vi "INR.vi"(1 "Port":refnum<visa-resource-name>="COM4" caption="VISA 리소스 이름", 2 "baud rate (9600)":u32=115200 caption="보 전송속도(9600)") -> (0 "InPOS (X)":bool, 3 "VISA out":refnum<visa-resource-name>, 4 "InPOS (Y)":bool, 5 "Limit+  (X)":bool, 6 "Limit+ (Y)":bool, 7 "Limit-  (X)":bool, 8 "Limit- (Y)":bool, 9 "HOMing  (X)":bool, 10 "HOMing(Y)":bool, 11 "RUN  (X)":bool, 12 "INR Information(X)":string, 13 "INR Information(Y)":string, 14 "Error Out":errorcluster caption="에러 출력", 15 "RUN (Y)":bool)   [LabVIEW 2010]
uses:
  <vilib>/Instr/_visa.llb/VISA Flush IO Buffer Mask.ctl
  <vilib>/Instr/_visa.llb/VISA Configure Serial Port (Instr).vi
panel:
  out "Status Y":bool[](array[boolean])
  out "Status X":bool[](array[boolean])
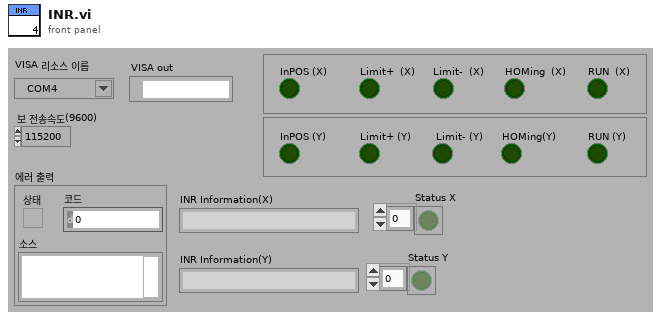
[diagram p1: front panel]
types:
  T1 = typedef "VISA Flush IO Buffer Mask.ctl" = u16
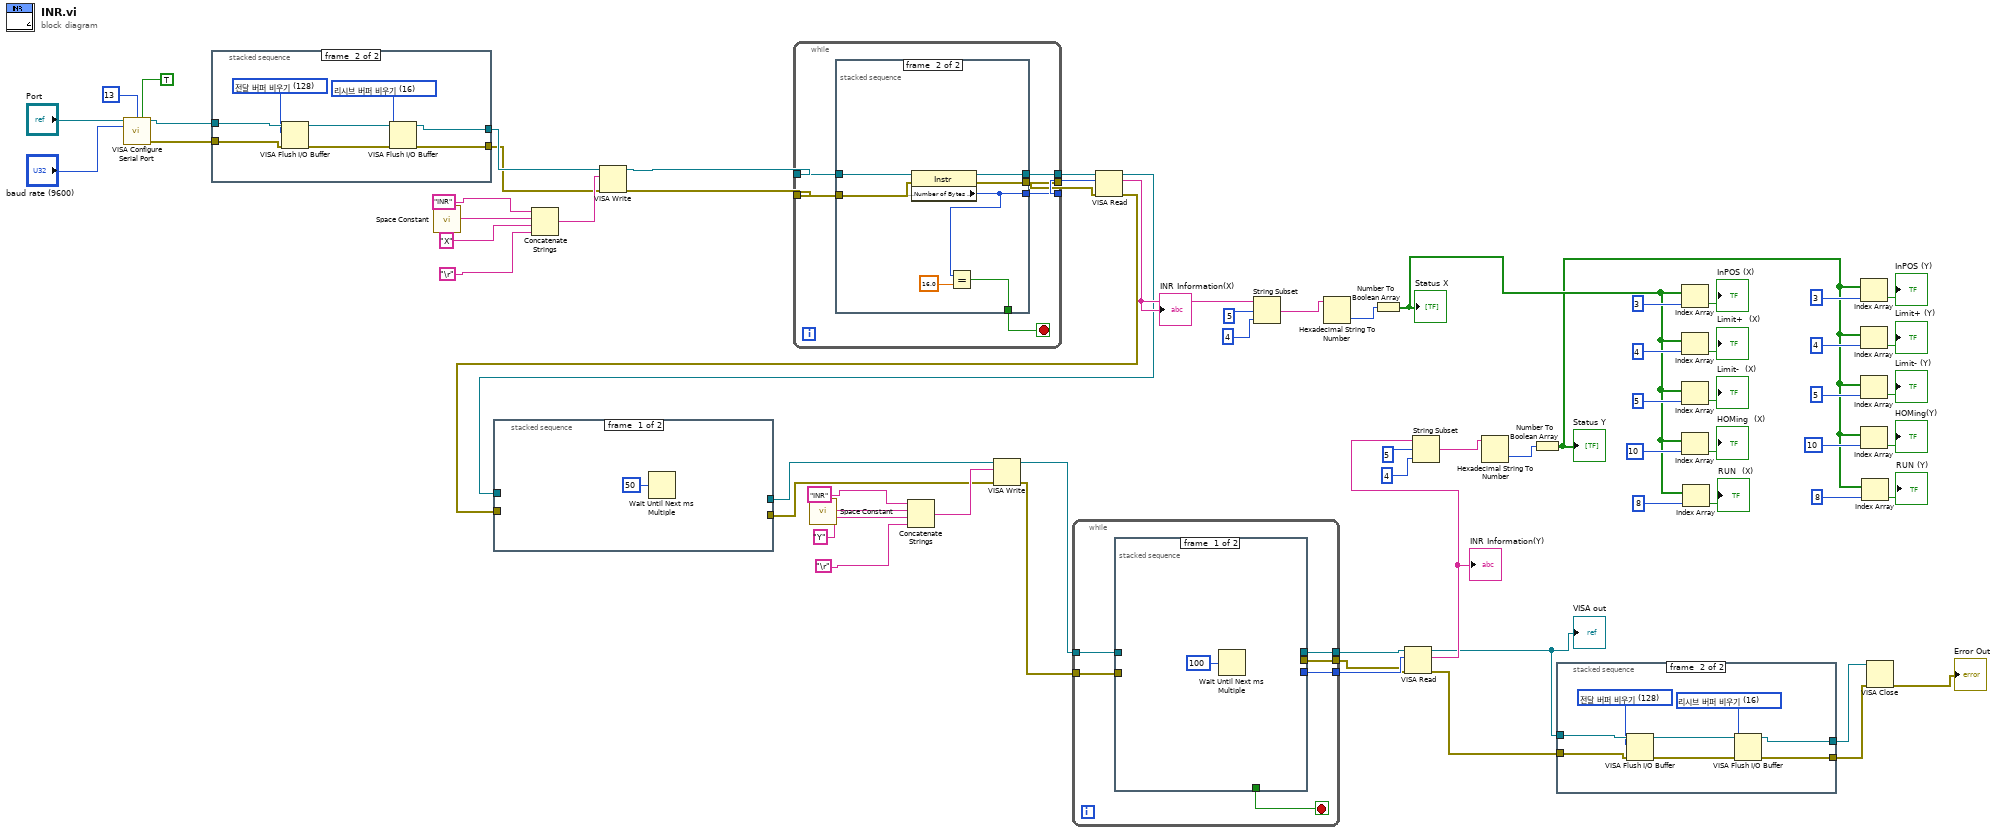
[diagram p0: block diagram]
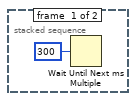
[diagram p2: hidden frame]
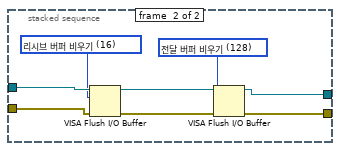
[diagram p3: hidden frame]
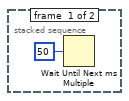
[diagram p4: hidden frame]
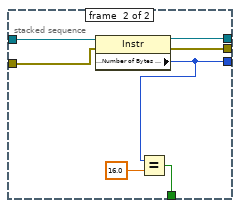
[diagram p5: hidden frame]
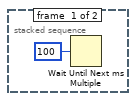
[diagram p6: hidden frame]
diagram:
  n1 = call-poly "VISA Configure Serial Port"("VISA resource name"="Port", "termination char\n(0xA = '\\n' = LF)"=i16 13 ("termination char\n(0xA = '\\n' = LF)"), "Enable Termination\nChar (T)"=TRUE ("Enable Termination\nChar (T)"), "baud rate (9600)"="baud rate (9600)") -> ("VISA resource name out"=w34:refnum<visa-resource-name>, "error out"=w33:errorcluster)  [unwired: 10 in]
  n2 = stacked-sequence {
    tunnel: w34 -> [_ w78]
    tunnel: w33 -> [_ w77]
    tunnel: [_ w73] -> w32
    tunnel: [_ w72] -> w31
    frame #0 {
      n3 = Wait Until Next ms Multiple(millisecond multiple=u32 50 ("ms 배수")) -> ()  [unwired: 1 out]
    }
    frame #1 {
      w71 = T1 16 items=["리시브 버퍼 비우기"=16, "전달 버퍼 디바이스에 쓰기"=32, "리시브 버퍼 비우기(I/O 없음)"=64, "전달 버퍼 비우기"=128] ("Mask")
      w76 = T1 128 items=["리시브 버퍼 비우기"=16, "전달 버퍼 디바이스에 쓰기"=32, "리시브 버퍼 비우기(I/O 없음)"=64, "전달 버퍼 비우기"=128] ("Mask")
      n4 = VISA Flush I/O Buffer(VISA resource name=w78, mask (16)=w76, error in (no error)=w77) -> (VISA resource name out=w75:refnum<visa-resource-name>, error out=w74:errorcluster)
      n5 = VISA Flush I/O Buffer(VISA resource name=w75, mask (16)=w71, error in (no error)=w74) -> (VISA resource name out=w73:refnum<visa-resource-name>, error out=w72:errorcluster)
    }
  }
  n6 = call <vilib>:"Space Constant.vi"() -> ("String"=w67:string)
  n7 = Concatenate Strings("INR", w67, "X", "\r") -> (w68:string)
  n8 = VISA Write(VISA resource name=w32, write buffer=w68, error in (no error)=w31) -> (VISA resource name out=w62:refnum<visa-resource-name>, error out=w61:errorcluster)  [unwired: 1 out]
  n9 = while {
    tunnel: w62 -> [w84]
    tunnel: w61 -> [w83]
    tunnel: [w82] -> w66
    tunnel: [w80] -> w65
    tunnel: [w81] -> w64
    stop <- w79 stop-if-true
    n10 = stacked-sequence {
      tunnel: w84 -> [_ w92]
      tunnel: w83 -> [_ w91]
      tunnel: [_ w90] -> w82
      tunnel: [_ w89] -> w81
      tunnel: [_ w87] -> w80
      tunnel: [_ w86] -> w79
      frame #0 {
        n11 = Wait Until Next ms Multiple(millisecond multiple=u32 100 ("대기 시간(ms)")) -> ()  [unwired: 1 out]
      }
      frame #1 {
        n12 = property class="Instr"(reference=w92, error in=w91) -> (reference out=w90:refnum<visa-resource-name>, error out=w89:errorcluster, "Serial Settings:Number of Bytes at Serial Port"=w87:u32)
        n13 = Equal?(x=w87, y=16.0) -> (x = y?=w86:bool)
      }
    }
  }
  n14 = call <vilib>:"Space Constant.vi"() -> ("String"=w59:string)
  n15 = Concatenate Strings("INR", w59, "Y", "\r") -> (w57:string)
  n16 = VISA Read(VISA resource name=w66, byte count=w65, error in (no error)=w64) -> (VISA resource name out=w28:refnum<visa-resource-name>, read buffer=w51:string, error out=w27:errorcluster)  [unwired: 1 out]
  "INR Information(X)" <- w51
  n17 = stacked-sequence {
    tunnel: w28 -> [_ w101]
    tunnel: w27 -> [_ w100]
    tunnel: [_ w96] -> w30
    tunnel: [_ w95] -> w29
    frame #0 {
      n18 = Wait Until Next ms Multiple(millisecond multiple=u32 50 ("ms 배수")) -> ()  [unwired: 1 out]
    }
    frame #1 {
      w94 = T1 128 items=["리시브 버퍼 비우기"=16, "전달 버퍼 디바이스에 쓰기"=32, "리시브 버퍼 비우기(I/O 없음)"=64, "전달 버퍼 비우기"=128] ("Mask")
      w99 = T1 16 items=["리시브 버퍼 비우기"=16, "전달 버퍼 디바이스에 쓰기"=32, "리시브 버퍼 비우기(I/O 없음)"=64, "전달 버퍼 비우기"=128] ("Mask")
      n19 = VISA Flush I/O Buffer(VISA resource name=w101, mask (16)=w99, error in (no error)=w100) -> (VISA resource name out=w98:refnum<visa-resource-name>, error out=w97:errorcluster)
      n20 = VISA Flush I/O Buffer(VISA resource name=w98, mask (16)=w94, error in (no error)=w97) -> (VISA resource name out=w96:refnum<visa-resource-name>, error out=w95:errorcluster)
    }
  }
  n21 = VISA Write(VISA resource name=w30, write buffer=w57, error in (no error)=w29) -> (VISA resource name out=w56:refnum<visa-resource-name>, error out=w55:errorcluster)  [unwired: 1 out]
  n22 = while {
    tunnel: w56 -> [w107]
    tunnel: w55 -> [w106]
    tunnel: [w105] -> w54
    tunnel: [w103] -> w53
    tunnel: [w104] -> w52
    stop <- w102 stop-if-true
    n23 = stacked-sequence {
      tunnel: w107 -> [_ w115]
      tunnel: w106 -> [_ w114]
      tunnel: [_ w113] -> w105
      tunnel: [_ w112] -> w104
      tunnel: [_ w110] -> w103
      tunnel: [_ w109] -> w102
      frame #0 {
        n24 = Wait Until Next ms Multiple(millisecond multiple=u32 100 ("대기 시간(ms)")) -> ()  [unwired: 1 out]
      }
      frame #1 {
        n25 = property class="Instr"(reference=w115, error in=w114) -> (reference out=w113:refnum<visa-resource-name>, error out=w112:errorcluster, "Serial Settings:Number of Bytes at Serial Port"=w110:u32)
        n26 = Equal?(x=w110, y=16.0) -> (x = y?=w109:bool)
      }
    }
  }
  n27 = String Subset(string=w51, offset (0)=5 ("오프셋(0)"), length (rest)=4 ("길이(나머지)")) -> (substring=w46:string)
  n28 = Hexadecimal String To Number(string=w46) -> (number=w45:u32)  [unwired: 2 in, 1 out]
  n29 = Number To Boolean Array(number=w45) -> (Boolean array=w12:bool[])
  "Status X" <- w12
  n30 = VISA Read(VISA resource name=w54, byte count=w53, error in (no error)=w52) -> (VISA resource name out=w26:refnum<visa-resource-name>, read buffer=w41:string, error out=w25:errorcluster)  [unwired: 1 out]
  "VISA out" <- w26
  "INR Information(Y)" <- w41
  n31 = String Subset(string=w41, offset (0)=5 ("오프셋(0)"), length (rest)=4 ("길이(나머지)")) -> (substring=w40:string)
  n32 = Hexadecimal String To Number(string=w40) -> (number=w42:u32)  [unwired: 2 in, 1 out]
  n33 = Number To Boolean Array(number=w42) -> (Boolean array=w1:bool[])
  "Status Y" <- w1
  n34 = stacked-sequence {
    tunnel: w26 -> [_ w124]
    tunnel: w25 -> [_ w123]
    tunnel: [_ w119] -> w24
    tunnel: [_ w118] -> w23
    frame #0 {
      n35 = Wait Until Next ms Multiple(millisecond multiple=u32 300 ("ms 배수")) -> ()  [unwired: 1 out]
    }
    frame #1 {
      w117 = T1 16 items=["리시브 버퍼 비우기"=16, "전달 버퍼 디바이스에 쓰기"=32, "리시브 버퍼 비우기(I/O 없음)"=64, "전달 버퍼 비우기"=128] ("Mask")
      w122 = T1 128 items=["리시브 버퍼 비우기"=16, "전달 버퍼 디바이스에 쓰기"=32, "리시브 버퍼 비우기(I/O 없음)"=64, "전달 버퍼 비우기"=128] ("Mask")
      n36 = VISA Flush I/O Buffer(VISA resource name=w124, mask (16)=w122, error in (no error)=w123) -> (VISA resource name out=w121:refnum<visa-resource-name>, error out=w120:errorcluster)
      n37 = VISA Flush I/O Buffer(VISA resource name=w121, mask (16)=w117, error in (no error)=w120) -> (VISA resource name out=w119:refnum<visa-resource-name>, error out=w118:errorcluster)
    }
  }
  n38 = Index Array(array=w12, index=3 ("인덱스")) -> (element=→"InPOS (X)":bool)
  n39 = Index Array(array=w12, index=4 ("인덱스")) -> (element=→"Limit+  (X)":bool)
  n40 = Index Array(array=w12, index=5 ("인덱스")) -> (element=→"Limit-  (X)":bool)
  n41 = Index Array(array=w12, index=10 ("인덱스")) -> (element=→"HOMing  (X)":bool)
  n42 = Index Array(array=w12, index=8 ("인덱스")) -> (element=→"RUN  (X)":bool)
  n43 = Index Array(array=w1, index=3 ("인덱스")) -> (element=→"InPOS (Y)":bool)
  n44 = Index Array(array=w1, index=4 ("인덱스")) -> (element=→"Limit+ (Y)":bool)
  n45 = Index Array(array=w1, index=5 ("인덱스")) -> (element=→"Limit- (Y)":bool)
  n46 = Index Array(array=w1, index=10 ("인덱스")) -> (element=→"HOMing(Y)":bool)
  n47 = Index Array(array=w1, index=8 ("인덱스")) -> (element=→"RUN (Y)":bool)
  n48 = VISA Close(VISA resource name=w24, error in (no error)=w23) -> (error out=→"Error Out":errorcluster)
